vi "Get Data.vi"(8 "error in":errorcluster, 11 "TSI 3025 in":refnum<class "TSI 3025.lvclass">) -> (0 "error out":errorcluster, 2 "Data Out":refnum<class "CPC Data.lvclass">, 3 "TSI 3025 out":refnum<class "TSI 3025.lvclass">)   [LabVIEW 2013, in "TSI 3025.lvclass"]
uses:
  TSI 3025.lvclass
  Data/CPC Data.lvclass
  CPC.lvclass
  Data/CPC Data.lvclass/CPC Data.ctl
  Data/Read Buffer Counts.vi
  Data/Write Buffer Counts.vi
  Read 200 s Buffer.vi
  Read 20 s Buffer.vi
  Read Optics T.vi
  Read Pump Value.vi
  Data/Read instrT.vi
  Data/Write instrT.vi
  Data/Write pumpV.vi
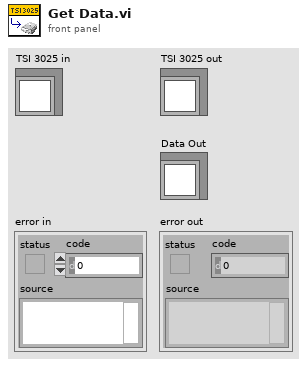
[diagram p1: front panel]
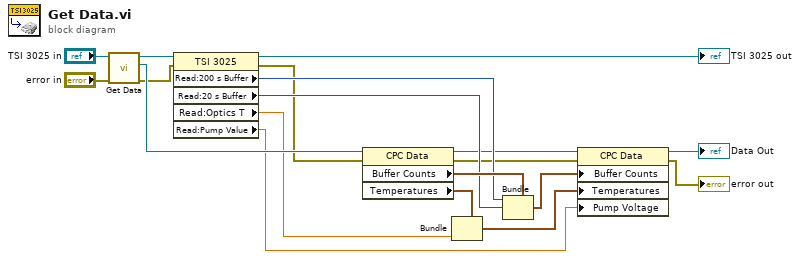
[diagram p0: block diagram]
diagram:
  n1 = call-parent "Get Data.vi"("error in"="error in", "CPC in"="TSI 3025 in") -> ("error out"=w11:errorcluster, "Data Out"=w16:refnum<class "CPC Data.lvclass">, "CPC out"=w17:refnum<class "TSI 3025.lvclass">)  [unwired: 7 in]
  n2 = property class="TSI 3025"(reference=w17, error in=w11) -> (reference out=→"TSI 3025 out":refnum<class "TSI 3025.lvclass">, error out=w5:errorcluster, "Read:200 s Buffer"=w14:i32, "Read:20 s Buffer"=w13:i32, "Read:Optics T"=w7:dbl, "Read:Pump Value"=w1:dbl)
  n3 = property class="CPC Data"(reference=w16, error in=w5) -> (reference out=w10:refnum<class "CPC Data.lvclass">, error out=w9:errorcluster, "Buffer Counts"=w15:cluster{"200 s":u32, "20 s":u32, "1 s":u32}, "Temperatures"=w8:cluster{"cond T":dbl, "sat T":dbl, "opt T":dbl})
  n4 = Bundle(cluster=w8, "opt T"=w7) -> (w6:cluster{"cond T":dbl, "sat T":dbl, "opt T":dbl})  [unwired: 2 in]
  n5 = Bundle(cluster=w15, "200 s"=w14, "20 s"=w13) -> (w12:cluster{"200 s":u32, "20 s":u32, "1 s":u32})  [unwired: 1 in]
  n6 = property class="CPC Data"(reference=w10, error in=w9, "Buffer Counts"=w12, "Temperatures"=w6, "Pump Voltage"=w1) -> (reference out=→"Data Out":refnum<class "CPC Data.lvclass">, error out=→"error out":errorcluster)
